vi "CRYRun State Manage.vi"(0 "Steps config.":bool[](array[boolean]), 5 "Pass?":bool, 7 "Last step?":bool, 11 "Seq setup flattened":string) -> (4 "Wait for confirmation":bool, 6 "Continue Sequence":bool)   [LabVIEW 2013]
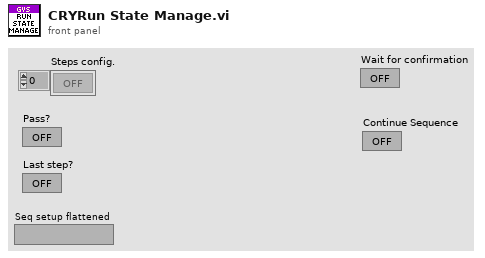
[diagram p1: front panel]
types:
  T1 = typedef "CRYStart Cluster.ctl" = cluster{"SequenceName":string, "Preload Stimulus":bool, "CloseOpenedDisplay":bool, "ClearMeasuredData":bool, "UpdateDisplayDuringRun":bool, "DisplayForConfirmation":bool, "HaltOnFail":bool, "UseSameHardware":bool, "UseSameCalibration":bool}
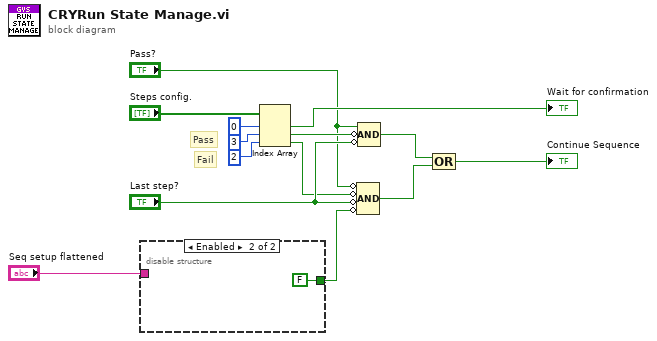
[diagram p0: block diagram]
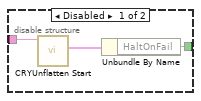
[diagram p2: hidden frame]
diagram:
  # "Pass"
  # "Fail"
  n1 = disable-structure shown="Enabled" {
    disable-tunnel: "Seq setup flattened" -> [w17 _]
    disable-tunnel: [w15 FALSE ("HaltOnFail")] -> w1
    frame Disabled {
      n2 = call "CRYUnflatten Start.vi"("Unflatten Sequence"=w17) -> ("Sequence Configure"=w16:T1)  [unwired: 8 in, 2 out]
      n3 = Unbundle By Name(w16) -> ("HaltOnFail"=w15:bool)
    }
    frame Enabled {
    }
  }
  n4 = Index Array(array="Steps config.", index #1=0 ("index"), index #2=3 ("index"), index #3=2 ("index")) -> (element #1=→"Wait for confirmation":bool, element #2=w11:bool, element #3=w8:bool)
  n5 = Compound Arithmetic op=AND(invert "Pass?", invert w8, invert "Last step?", invert w1) -> (w5:bool)
  n6 = Compound Arithmetic op=AND("Pass?", invert w11, invert "Last step?") -> (w6:bool)
  n7 = Compound Arithmetic op=OR(w6, w5) -> (→"Continue Sequence":bool)
